vi "Test Deserialize Null To Defaults.vi"(8 "error in (no error)":errorcluster) -> (0 "error out":errorcluster)   [LabVIEW 2013]
uses:
  <vilib>/addons/_JKI Toolkits/Caraya/classes/Test/Test.lvclass
  src/JKI JSON Serialization.lvlib
  <vilib>/addons/_JKI Toolkits/Caraya/classes/Assert/Assert.lvclass
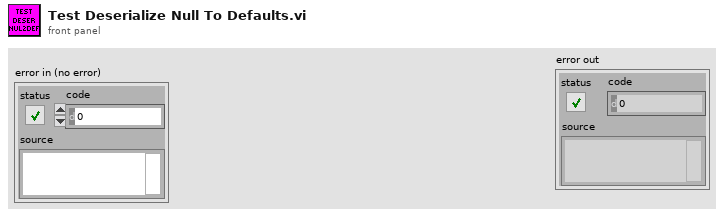
[diagram p1: front panel]
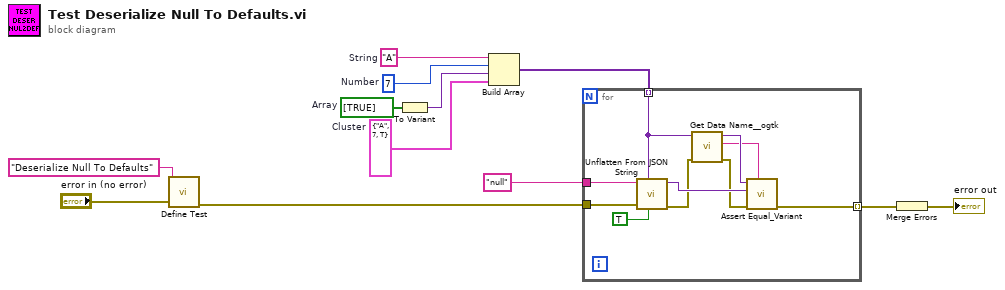
[diagram p0: block diagram]
diagram:
  w3 = cluster{"String":string, "Number":i32, bool} {"String"="A", "Number"=7, TRUE}  # Cluster
  w4 = bool[] [TRUE]  # Array
  w5 = 7  # Number
  w1 = "A"  # String
  n1 = call <vilib>:"Define Test.vi"("error in (no error)"="error in (no error)", "Label (VI Title)"="Deserialize Null To Defaults") -> ("error out"=w7:errorcluster)  [unwired: 9 in]
  n2 = To Variant(anything=w4) -> (Variant=w2:variant)
  n3 = Build Array(w1, w5, w2, w3) -> (w6:variant[])
  n4 = for {
    tunnel: "null" ("JSON String") -> [w22]
    tunnel: [w15] -> w8 mode=indexing
    tunnel: w7 -> [w14]
    tunnel: w6 -> [w13] mode=indexing
    n5 = call "Unflatten From JSON String.vi"("Nulls as Defaults (T)"=TRUE, "Type and Defaults"=w13, "error in (no error)"=w14, "JSON String"=w22) -> ("error out"=w17:errorcluster, "Variant"=w20:variant)  [unwired: 6 in]
    n6 = call <userlib>:"Get Data Name__ogtk.vi"("error in (no error)"=w17, "Data"=w13) -> ("error out"=w16:errorcluster, "Data Name"=w18:string, "Data dup"=w19:variant)  [unwired: 7 in]
    n7 = call <vilib>:"Assert Equal_Variant.vi"("Label"=w18, "error in (no error)"=w16, "Y"=w20, "X"=w19) -> ("error out"=w15:errorcluster)  [unwired: 7 in]
  }
  n8 = Merge Errors(w8) -> (→"error out":errorcluster)
